vi "ModuleSelectItem.vi"(10 "TestModel":string, 11 "Module select":refnum<vi>) -> (2 "InitSelect":string, 3 "ViPathOut":path, 4 "PassYeildHistory":dbl[](array[numeric]) format="%0.3f")   [LabVIEW 2013]
uses:
  <vilib>/Utility/file.llb/Read From Spreadsheet File (DBL).vi
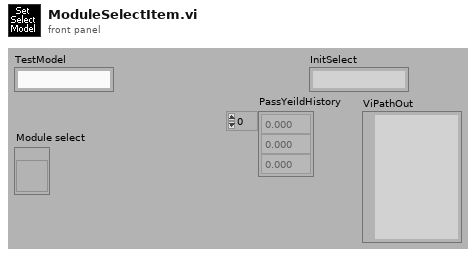
[diagram p1: front panel]
types:
  T1 = enum32{"invalid app kind", "Development System", "Run Time System", "Student Edition", "Embedded LabVIEW", "Evaluation", "Custom"}
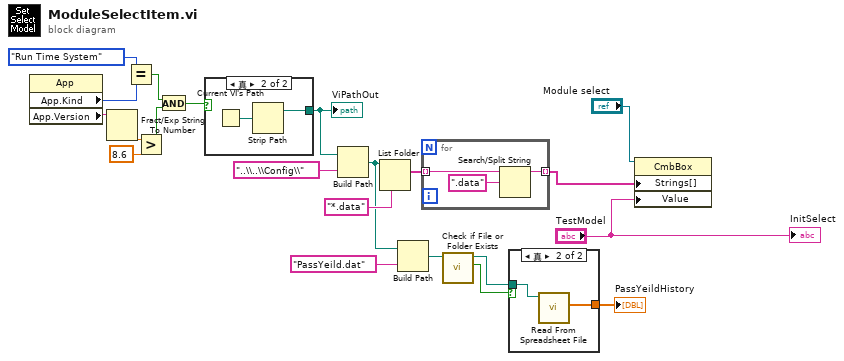
[diagram p0: block diagram]
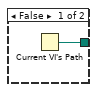
[diagram p2: hidden frame]
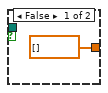
[diagram p3: hidden frame]
diagram:
  n1 = property class="App"() -> ("App.Kind"=w9:T1, "App.Version"=w8:string)  [unwired: 2 in, 2 out]
  n2 = Fract/Exp String To Number(string=w8) -> (number=w7:dbl)  [unwired: 4 out]
  n3 = Equal?(x=T1."Run Time System" ("y"), y=w9) -> (x = y?=w5:bool)
  n4 = Greater?(x=w7, y=8.6) -> (0:w4:bool)
  n5 = And(x=w5, y=w4) -> (x .and. y?=w3:bool)
  n6 = case shown="真" w3 {
    tunnel: [w22 w24] -> w2
    frame False {
      n7 = Current VI's Path() -> (path=w22:path)
    }
    frame True {
      n8 = Current VI's Path() -> (path=w23:path)
      n9 = Strip Path(path=w23) -> (stripped path=w24:path)  [unwired: 1 out]
    }
  }
  "ViPathOut" <- w2
  n10 = Build Path(base path=w2, name or relative path="..\\..\\Config\\" ("名称或相对路径")) -> (appended path=w1:path)
  n11 = List Folder(path=w1, pattern="*.data") -> (filenames=w21:string[])  [unwired: 1 in, 4 out]
  n12 = Build Path(base path=w1, name or relative path="PassYeild.dat" ("pattern")) -> (appended path=w14:path)
  n13 = for {
    tunnel: w21 -> [w26] mode=indexing
    tunnel: [w25] -> w18 mode=indexing
    n14 = Search/Split String(string=w26, search string/char (-)=".data" ("搜索字符串/字符(-)")) -> (substring before match=w25:string)  [unwired: 3 out]
  }
  n15 = call <vilib>:"Check if File or Folder Exists.vi"("path"=w14) -> ("file or folder exists?"=w15:bool, "dup path"=w13:path)  [unwired: 1 in, 8 out]
  n16 = case shown="真" w15 {
    tunnel: w13 -> [_ w30]
    tunnel: [dbl[] [] ("first row") w29] -> w12
    frame False {
    }
    frame True {
      n17 = call-poly <vilib>:"Read From Spreadsheet File.vi"("file path (dialog if empty)"=w30) -> ("first row"=w29:dbl[])  [unwired: 3 in, 7 out]
    }
  }
  "PassYeildHistory" <- w12
  n18 = property class="CmbBox"(reference="Module select", "Strings[]"=w18, "Value"="TestModel") -> ()  [unwired: 1 in, 2 out]
  "InitSelect" <- "TestModel"
